vi "Stop task.vi"(4 "error in":errorcluster, 5 "input main cluster":T1, 7 "index":i32) -> (0 "error out":errorcluster, 1 "output main cluster":T1)   [LabVIEW 2010]
uses:
  Main_cluster.ctl
  <vilib>/vision/Image Controls.llb/IMAQ Image.ctl
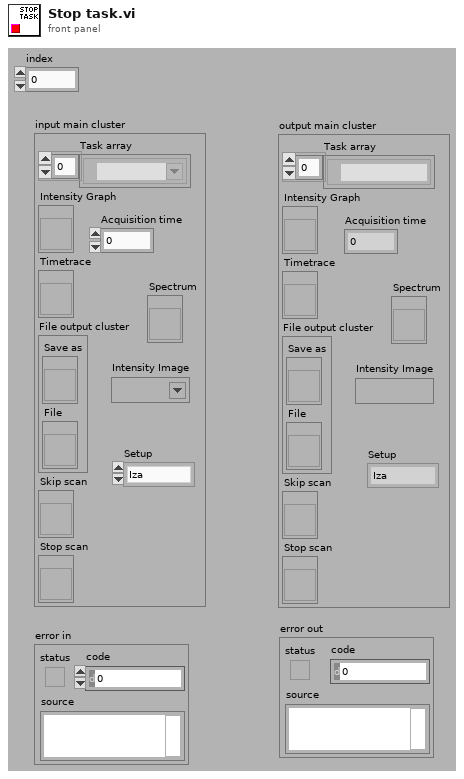
[diagram p1: front panel]
types:
  T1 = typedef "Main_cluster.ctl" = cluster{"Task array":refnum<k21>[], "Intensity Graph":refnum<vi>, "Timetrace":refnum<vi>, "File output cluster":cluster{"Save as":refnum<vi>, "File":refnum<vi>}, "Skip scan":refnum<vi>, "Stop scan":refnum<vi>, "Acquisition time":dbl, "Setup":enum16{"Iza", "Lukasz"}, "Spectrum":refnum<vi>, "Intensity Image":T2}
  T2 = typedef "IMAQ Image.ctl" = refnum<image>
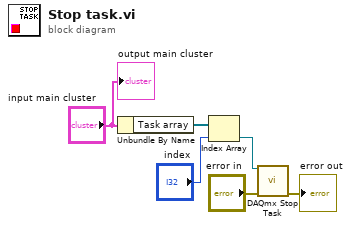
[diagram p0: block diagram]
diagram:
  n1 = Unbundle By Name("input main cluster") -> ("Task array"=w2:refnum<k21>[])
  n2 = Index Array(array=w2, index="index") -> (element=w4:refnum<k21>)
  n3 = call <vilib>:"DAQmx Stop Task.vi"("task/channels in"=w4, "error in"="error in") -> ("error out"=→"error out":errorcluster)  [unwired: 13 out]
  "output main cluster" <- "input main cluster"
